vi "Read.vi"(8 "error in (no error)":errorcluster, 11 "CVT_String in":refnum<class "CVT_String.lvclass">) -> (0 "error out":errorcluster, 2 "value":string, 3 "CVT_String out":refnum<class "CVT_String.lvclass">)   [LabVIEW 2024, in "Current Value Table.lvlib" / "CVT_String.lvclass"]
uses:
  CVT_String.lvclass
  CVT_String.lvclass/CVT_String.ctl
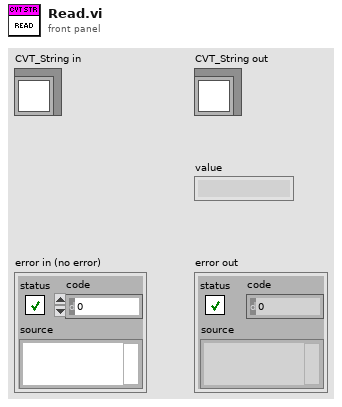
[diagram p1: front panel]
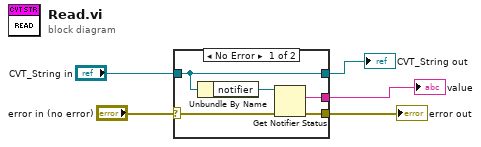
[diagram p0: block diagram]
diagram:
  n1 = case shown="No Error" "error in (no error)" {
    selector: "error in (no error)" -> [w7 w12]
    tunnel: [w6 w12] -> w4
    tunnel: [w10 w11] -> w2
    tunnel: "CVT_String in" -> [w10 w11]
    tunnel: [w8 _] -> w1
    frame No Error {
      n2 = Unbundle By Name(w10) -> ("notifier"=w9:refnum<notifier>)
      n3 = Get Notifier Status(notifier=w9, error in (no error)=w7) -> (current notification=w8:string, error out=w6:errorcluster)  [unwired: 3 out]
    }
    frame Error {
    }
  }
  "error out" <- w4
  "CVT_String out" <- w2
  "value" <- w1
